vi "StartStop Device.vi"(6 "parseError? T:Yes":bool=TRUE, 8 "error in (no error)":errorcluster, 10 "Start/Stop (f:Stop)":bool, 11 "VISA resource name":refnum<visa-resource-name>) -> (0 "error out":errorcluster, 3 "VISA resource name out":refnum<visa-resource-name>)   [LabVIEW 2015, in "JULABO DeviceDriver.lvlib"]
doc: "This VI starts the instrument (<B>true</B>) or stops it (<B>false</B>)"
uses:
  JULABO DeviceDriver.lvlib
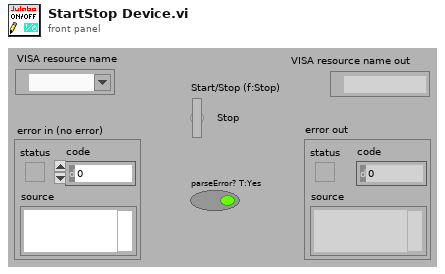
[diagram p1: front panel]
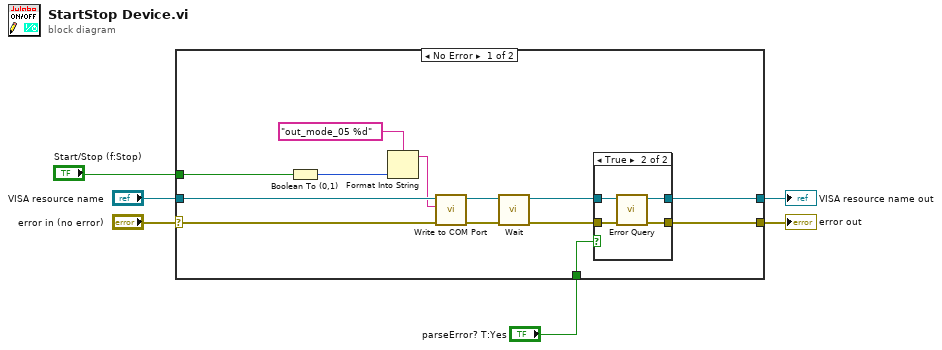
[diagram p0: block diagram]
diagram:
  n1 = case shown="No Error" "error in (no error)" {
    selector: "error in (no error)" -> [w18 w26]
    tunnel: "VISA resource name" -> [w19 w27]
    tunnel: [w16 w26] -> w5
    tunnel: [w15 w27] -> w4
    tunnel: "Start/Stop (f:Stop)" -> [w17 _]
    tunnel: "parseError? T:Yes" -> [w14 _]
    frame No Error {
      n2 = Boolean To (0,1)(Boolean=w17) -> (0, 1=w7:i16)
      n3 = Format Into String(format string="out_mode_05 %d", w7) -> (resulting string=w8:string)  [unwired: 2 in, 1 out]
      n4 = call "Write to COM Port.vi"("error in"=w18, "Command (input)"=w8, "VISA resource name in"=w19) -> ("error out"=w12:errorcluster, "VISA resource name out"=w13:refnum<visa-resource-name>)  [unwired: 7 in]
      n5 = call "Wait.vi"("error in"=w12, "VISA resource name in"=w13) -> ("error out"=w10:errorcluster, "VISA resource name out"=w11:refnum<visa-resource-name>)  [unwired: 4 in]
      n6 = case shown="True" w14 {
        tunnel: w11 -> [w21 w25]
        tunnel: w10 -> [w20 w24]
        tunnel: [w21 w23] -> w15
        tunnel: [w20 w22] -> w16
        frame False {
        }
        frame True {
          n7 = call "Error Query.vi"("error in (no error)"=w24, "VISA resource name"=w25) -> ("error out"=w22:errorcluster, "VISA resource name out"=w23:refnum<visa-resource-name>)  [unwired: 6 in, 2 out]
        }
      }
    }
    frame Error {
    }
  }
  "error out" <- w5
  "VISA resource name out" <- w4
